vi "read_single_dat_file.vi"() -> ()   [LabVIEW 2019]
uses:
  ee0b76d9-a073-48a3-95c3-88ad152f60d4.vi
  <vilib>/Analysis/3filter.llb/Equi-Ripple LowPass (DBL).vi
  <instrlib>/niRFSA/niRFSA.llb/niRFSA Get IQ Components (Complex Cluster).vi
  <vilib>/Analysis/NI_AALBase.lvlib
panel:
  in  "Remove Frequency Offset":bool
  out "Amplitude Stability":dbl format="%.6p"
  in  "Low Pass Filter  (To remove noise, only works if the signal is close to baseband)":T1={"Enable"=FALSE, "Pass Band"=20000.0, "Stop Band"=40000.0} {"Stop Band" format="%.6p"; "Pass Band" format="%.6p"}
  out "Phase Stability":dbl format="%.6p"
  in  "Sample Rate":dbl=5000000.0 format="%.6p"
  in  "Tab Control":enum32{"IQ", "Magnitude", "Phase"}(tab)
  out "IQ":cluster{"t0":dbl, "dt":dbl, "Y":dbl[]}[](graph)
  out "Magnitude":cluster{"to":dbl, "dt":dbl, "Y":dbl[]}(graph)
  out "Phase":cluster{"t0":dbl, "dt":dbl, "Y":dbl[]}(graph)
  in  "offset (in bytes) (0)":i64
  in  "count (elements)":i32=8192
  in  "file path (use dialog)":path=path "C:/_Opps/20200310-David/read_dat_file/txrxrx_n321_rate5e6_lo_cw500e6_march10_500pm.00.dat"
  out "error out":errorcluster
  # "set to -1 to read the whole file"
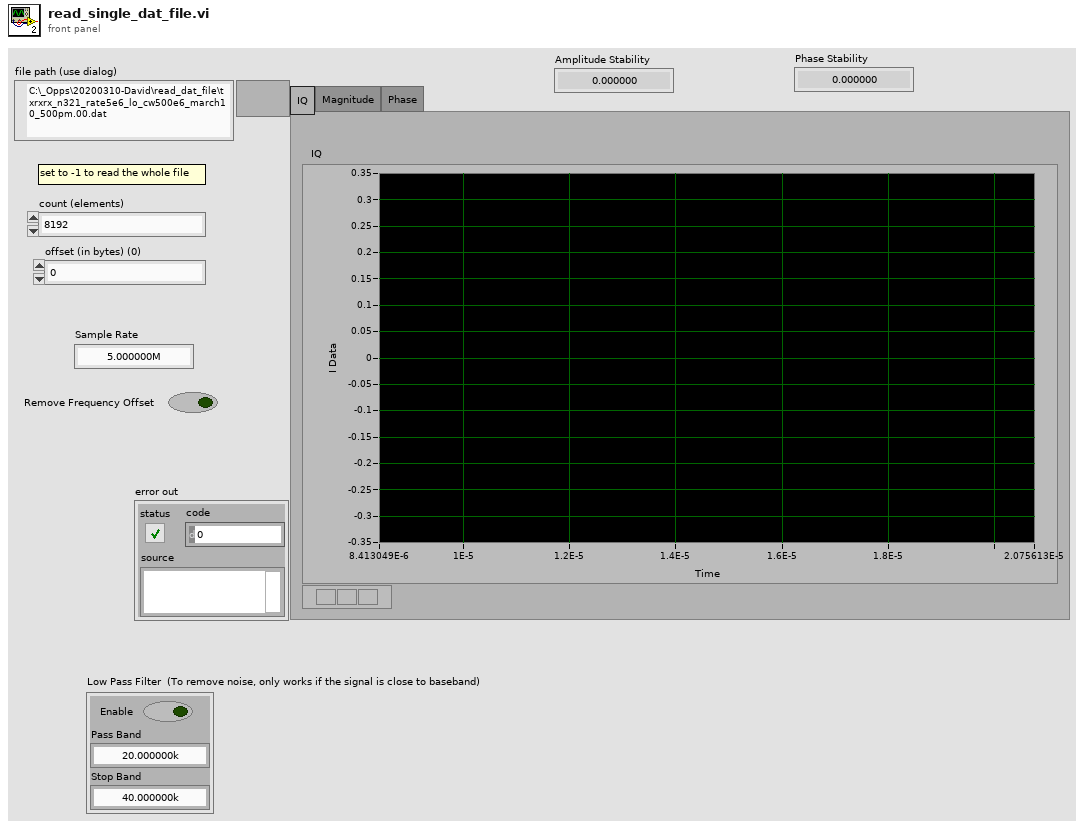
[diagram p1: front panel]
types:
  T1 = cluster{"Enable":bool, "Pass Band":dbl, "Stop Band":dbl}
  T2 = enum16{"open", "replace", "create", "open or create", "replace or create", "replace or create with confirmation"}
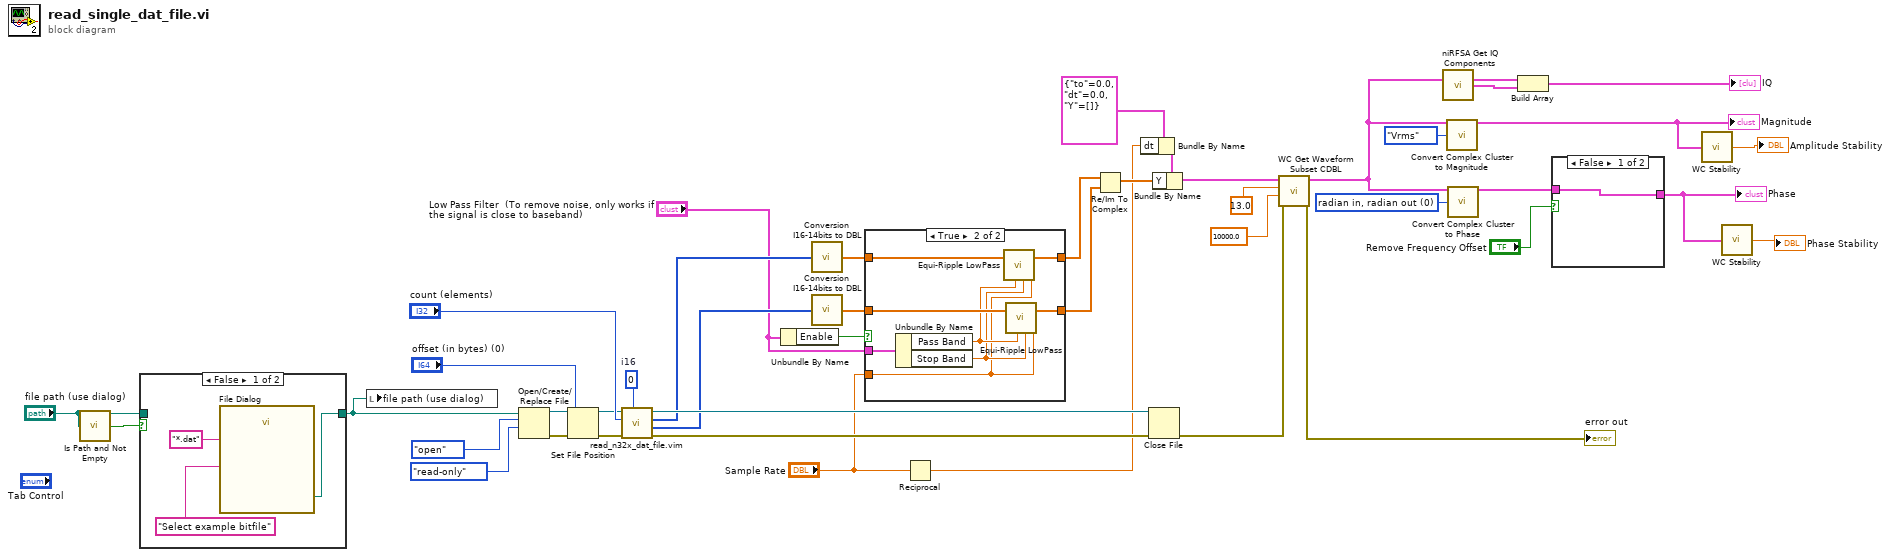
[diagram p0: block diagram]
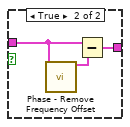
[diagram p2: hidden frame]
diagram:
  w16 = 0 items=["radian in, radian out", "radian in, degree out", "degree in, degree out", "degree in, radian out"] ("phase unit")
  w34 = i16 0  # i16
  n1 = call <vilib>:"Is Path and Not Empty.vi"("path"="file path (use dialog)") -> ("Is Path and Not Empty?"=w33:bool)  [unwired: 4 in]
  n2 = case shown="False" w33 {
    tunnel: "file path (use dialog)" -> [_ w48]
    tunnel: [w46 w48] -> w31
    frame False {
      n3 = call "File Dialog"("prompt"="Select example bitfile", "pattern (all files)"="*.dat") -> ("selected path"=w46:path)  [unwired: 10 in, 3 out]
    }
    frame True {
    }
  }
  n4 = local write "file path (use dialog)"(w31) -> ()
  n5 = Open/Create/Replace File(file path (use dialog)=w31, operation (0:open)=T2."open", access (0:read/write)=enum16{"read/write", "read-only", "write-only"}."read-only") -> (refnum out=w39:refnum<file>, error out=w38:errorcluster)  [unwired: 3 in, 1 out]
  n6 = Set File Position(offset (in bytes) (0)="offset (in bytes) (0)", refnum=w39, error in=w38) -> (refnum out=w36:refnum<file>, error out=w35:errorcluster)  [unwired: 1 in]
  n7 = call "read_n32x_dat_file.vim"("type"=w34, "error in"=w35, "count"="count (elements)", "file refnum in"=w36) -> ("error out"=w41:errorcluster, "Q Data"=w29:i16[], "I Data"=w30:i16[], "file refnum out"=w42:refnum<file>)  [unwired: 3 in, 1 out]
  n8 = Unbundle By Name("Low Pass Filter  (To remove noise, only works if the signal is close to baseband)") -> ("Enable"=w25:bool)
  n9 = call "Conversion I16-14bits to DBL.vi"("Array"=w30) -> ("Array Out"=w27:dbl[])  [unwired: 4 in]
  n10 = call "Conversion I16-14bits to DBL.vi"("Array"=w29) -> ("Array Out"=w28:dbl[])  [unwired: 4 in]
  n11 = case shown="True" w25 {
    tunnel: w28 -> [w49 w58]
    tunnel: [w49 w57] -> w22
    tunnel: w27 -> [w50 w56]
    tunnel: [w50 w55] -> w23
    tunnel: "Sample Rate" -> [_ w52]
    tunnel: "Low Pass Filter  (To remove noise, only works if the signal is close to baseband)" -> [_ w51]
    frame False {
    }
    frame True {
      n12 = Unbundle By Name(w51) -> ("Pass Band"=w54:dbl, "Stop Band"=w53:dbl)
      n13 = call-poly <vilib>:"Equi-Ripple LowPass.vi"("pass freq"=w54, "stop freq"=w53, "sampling freq: fs"=w52, "X"=w56) -> ("Filtered X"=w55:dbl[])  [unwired: 2 in, 1 out]
      n14 = call-poly <vilib>:"Equi-Ripple LowPass.vi"("pass freq"=w54, "stop freq"=w53, "sampling freq: fs"=w52, "X"=w58) -> ("Filtered X"=w57:dbl[])  [unwired: 2 in, 1 out]
    }
  }
  n15 = Reciprocal(x="Sample Rate") -> (1/x=w19:dbl)
  n16 = Re/Im To Complex(1:w22, 2:w23) -> (0:w21:cdb[])
  n17 = Bundle By Name(cluster=cluster{"to":dbl, "dt":dbl, "Y":cdb[]} {"to"=0.0, "dt"=0.0, "Y"=[]} ("Cluster"), "dt"=w19) -> (w18:cluster{"to":dbl, "dt":dbl, "Y":cdb[]})
  n18 = Close File(refnum=w42, error in=w41) -> (error out=w4:errorcluster)  [unwired: 1 out]
  n19 = Bundle By Name(cluster=w18, "Y"=w21) -> (w12:cluster{"to":dbl, "dt":dbl, "Y":cdb[]})
  n20 = call "WC Get Waveform Subset CDBL.vi"("error in (no error)"=w4, "duration"=10000.0, "start samples/time"=13.0, "Waveform In"=w12) -> ("error out"=→"error out":errorcluster, "Waveform Out"=w11:cluster{"t0":dbl, "dt":dbl, "Y":cdb[]})  [unwired: 2 in, 2 out]
  n21 = call-poly <instrlib>:"niRFSA Get IQ Components.vi"("data"=w11) -> ("I"=w15:cluster{"t0":dbl, "dt":dbl, "Y":dbl[]}, "Q"=w14:cluster{"t0":dbl, "dt":dbl, "Y":dbl[]})  [unwired: 1 in, 12 out]
  n22 = call "Convert Complex Cluster to Magnitude.vi"("IQ data (complex) In"=w11, "Public.Units"=enum8{"Vrms", "dBm"}."Vrms") -> ("Magnitude Out"=w7:cluster{"t0":dbl, "dt":dbl, "Y":dbl[]})  [unwired: 12 in, 1 out]
  "Magnitude" <- w7
  n23 = call "Convert Complex Cluster to Phase.vi"("IQ data (complex) In"=w11, "phase unit"=w16) -> ("Phase Out"=w10:cluster{"t0":dbl, "dt":dbl, "Y":dbl[]})  [unwired: 12 in, 1 out]
  n24 = Build Array(w15, w14) -> (→"IQ":cluster{"t0":dbl, "dt":dbl, "Y":dbl[]}[])
  n25 = case shown="False" "Remove Frequency Offset" {
    tunnel: w10 -> [w59 w61]
    tunnel: [w59 w60] -> w9
    frame False {
    }
    frame True {
      n26 = call "Phase - Remove Frequency Offset.vi"("Phase In"=w61) -> ("Phase Out"=w62:cluster{"t0":dbl, "dt":dbl, "Y":dbl[]})  [unwired: 13 in, 1 out]
      n27 = Subtract(x=w61, y=w62) -> (x-y=w60:cluster{"t0":dbl, "dt":dbl, "Y":dbl[]})
    }
  }
  "Phase" <- w9
  n28 = call "WC Stability.vi"("Data In"=w7) -> ("Stability"=→"Amplitude Stability":dbl)  [unwired: 4 in]
  n29 = call "WC Stability.vi"("Data In"=w9) -> ("Stability"=→"Phase Stability":dbl)  [unwired: 4 in]
